vi "Jones_Manual_Rudder.vi"(0 "Full Port":bool, 1 "Port":bool, 2 "Starboard":bool, 3 "Full Starboard":bool, 4 "Array":dbl[](array[numeric])) -> (6 "Array 2":dbl[](array[numeric]))   [LabVIEW 2011]
panel:
  # "This control is passed an array"
  # "This indicator shows the output"
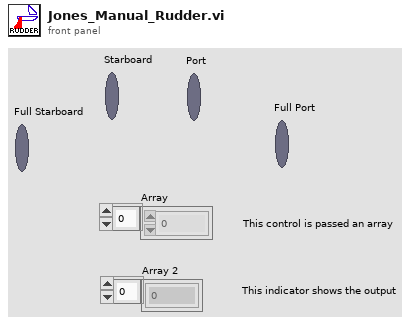
[diagram p1: front panel]
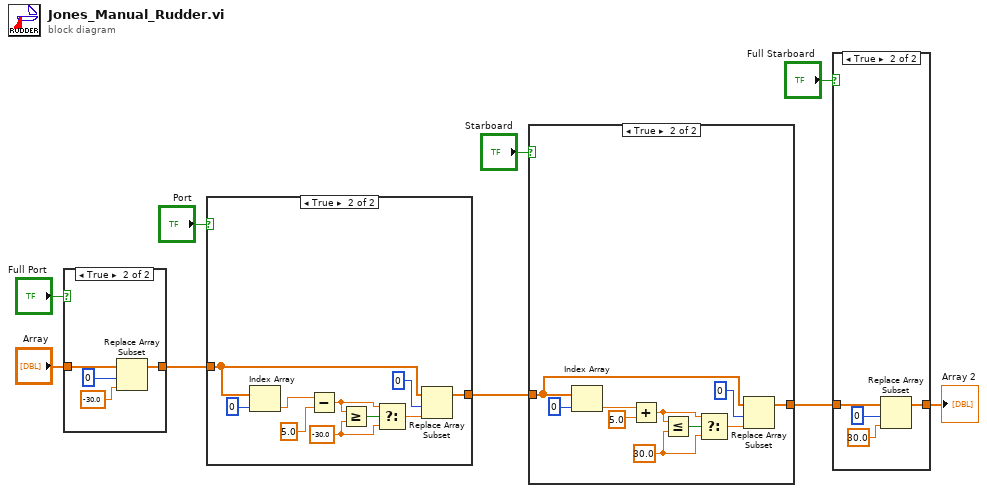
[diagram p0: block diagram]
diagram:
  n1 = case shown="True" "Full Port" {
    tunnel: "Array" -> [w10 w12]
    tunnel: [w10 w14] -> w7
    frame False {
    }
    frame True {
      n2 = Replace Array Subset(array=w12, new element=-30.0 ("new element/subarray"), index=0) -> (w14:dbl[])
    }
  }
  n3 = case shown="True" "Port" {
    tunnel: w7 -> [w15 w24]
    tunnel: [w15 w25] -> w5
    frame False {
    }
    frame True {
      w18 = -30.0
      n4 = Index Array(array=w24, index=0) -> (element=w17:dbl)
      n5 = Subtract(x=w17, y=5.0) -> (x-y=w20:dbl)
      n6 = Greater Or Equal?(x=w20, y=w18) -> (x >= y?=w21:bool)
      n7 = Select(t=w20, s=w21, f=w18) -> (s? t:f=w19:dbl)
      n8 = Replace Array Subset(array=w24, new element=w19, index=0) -> (w25:dbl[])
    }
  }
  n9 = case shown="True" "Starboard" {
    tunnel: w5 -> [w26 w35]
    tunnel: [w26 w36] -> w3
    frame False {
    }
    frame True {
      w30 = 30.0
      n10 = Index Array(array=w35, index=0) -> (element=w27:dbl)
      n11 = Add(x=w27, y=5.0 ("x")) -> (x+y=w28:dbl)
      n12 = Less Or Equal?(x=w28, y=w30) -> (x <= y?=w31:bool)
      n13 = Select(t=w28, s=w31, f=w30) -> (s? t:f=w32:dbl)
      n14 = Replace Array Subset(array=w35, new element=w32, index=0) -> (w36:dbl[])
    }
  }
  n15 = case shown="True" "Full Starboard" {
    tunnel: w3 -> [w37 w41]
    tunnel: [w37 w39] -> w2
    frame False {
    }
    frame True {
      n16 = Replace Array Subset(array=w41, new element=30.0 ("new element/subarray"), index=0) -> (w39:dbl[])
    }
  }
  "Array 2" <- w2
